vi "Pad Start and End.vi"(1 "Waveform":waveform(dbl)={"t0"=timestamp(3461330237.7970004 s since 1904-01-01), "dt"=1.0, "Y"=[9.0, 10.0, 10.5, 10.0, 8.5]}) -> (0 "Padded waveform":waveform(dbl)={"t0"=timestamp(3461330237.7970004 s since 1904-01-01), "dt"=1.0, "Y"=[9.0, 9.0, 9.0, 9.0, 9.0, 9.0, 10.0, 10.5, 10.0, 8.5, 8.5, 8.5, 8.5, 8.5, 8.5]})   [LabVIEW 2010]
panel:
  out "XY Graph":cluster{"X array":dbl[], "Y array":dbl[]}(graph)={"X array"=[0.0, 1.0, 2.0, 3.0, 4.0, 5.0, 6.0, 7.0, 8.0, 9.0, 10.0, 11.0, 12.0, 13.0, 14.0], "Y array"=[9.0, 9.0, 9.0, 9.0, 9.0, 9.0, 10.0, 10.5, 10.0, 8.5, 8.5, 8.5, 8.5, 8.5, 8.5]}
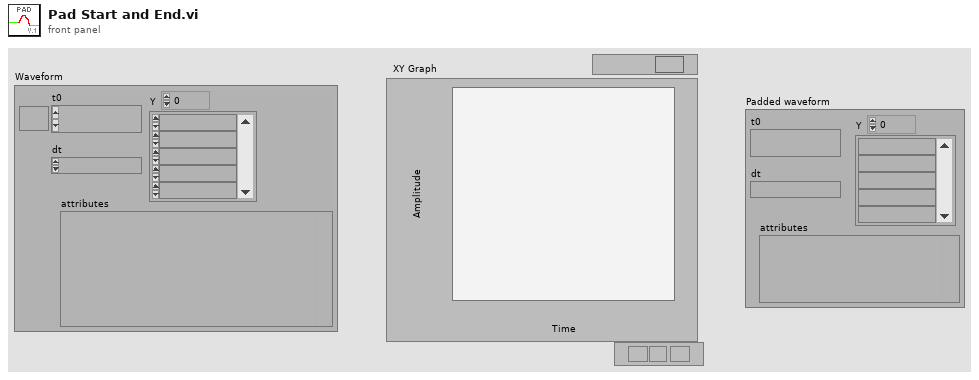
[diagram p1: front panel]
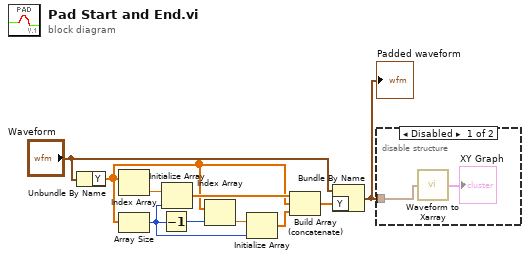
[diagram p0: block diagram]
diagram:
  n1 = Unbundle By Name("Waveform") -> ("Y"=w3:dbl[])
  n2 = Index Array(array=w3) -> (element=w8:dbl)  [unwired: 1 in]
  n3 = Array Size(array=w3) -> (size(s)=w2:i32)
  n4 = Decrement(x=w2) -> (x-1=w6:i32)
  n5 = Initialize Array(w8, w2) -> (w5:dbl[])
  n6 = Index Array(array=w3, index=w6) -> (element=w7:dbl)
  n7 = Initialize Array(w7, w2) -> (w4:dbl[])
  n8 = Build Array (concatenate)(w5, w3, w4) -> (w1:dbl[])
  n9 = Bundle By Name(cluster="Waveform", "Y"=w1) -> (w9:waveform(dbl))
  "Padded waveform" <- w9
  n10 = disable-structure shown="Disabled" {
    disable-tunnel: w9 -> [w12 _]
    frame Disabled {
      n11 = call "Waveform to Xarray.vi"("Waveform In"=w12) -> ("Single Plot"=→"XY Graph":cluster{"X array":dbl[], "Y array":dbl[]})
    }
    frame Enabled {
    }
  }
